vi "Write Image Header.vi"(8 "error in (no error)":errorcluster, 11 "Save Image in":refnum<class "Save Image.lvclass">) -> (0 "error out":errorcluster, 3 "Save Image out":refnum<class "Save Image.lvclass">)   [LabVIEW 2018, in "Save Image.lvclass"]
uses:
  Save Image.lvclass
  Save Image.lvclass/Save Image.ctl
  <userlib>/gfitsio/gfitsio-write-key-string.vi
  <userlib>/gfitsio/gfitsio.lvlib
  Simulated_Header/Simulated_Header.lvclass
panel:
  out "Header Contents":T1={"Header Content"={"FILENAME"={"Name"="FILENAME", "Value"="", "Comment"="File name at acquisition"}, "OBSERVER"={"Name"="OBSERVER", "Value"="", "Comment"="Name of the observer"}, "PROGRID"={"Name"="PROGRID", "Value"="", "Comment"="Program ID"}, "OBJECT"={"Name"="OBJECT", "Value"="", "Comment"="Object name"}, "NIGHTDIR"={"Name"="NIGHTDIR", "Value"="", "Comment"="Night directory name "}, "CHANNEL"={"Name"="CHANNEL", "Value"="", "Comment"="Instrument channel"}, "INSTRUME"={"Name"="INSTRUME", "Value"="", "Comment"="Instrument"}, "NEXPSEQ"={"Name"="NEXPSEQ", "Value"="", "Comment"="Total number of exposures in sequence"}, "SEQINDEX"={"Name"="SEQINDEX", "Value"="", "Comment"="Exposure index in the sequence"}, "OBSTYPE"={"Name"="OBSTYPE", "Value"="", "Comment"="Image type: OBJECT, BIAS, FLAT, ARC, DARK"}, "READMOD"={"Name"="READMOD", "Value"="", "Comment"="Read out mode: fast, normal, slow"}, "READMODE"={"Name"="READMODE", "Value"="", "Comment"="CCD read mode"}, "ACQMODE"={"Name"="ACQMODE", "Value"="", "Comment"="Acquisition Mode"}, "PREAMP"={"Name"="PREAMP", "Value"="", "Comment"="Pre-amplifier gain"}, "READOUT"={"Name"="READOUT", "Value"="", "Comment"="Readout Rate"}, "VSHIFT"={"Name"="VSHIFT", "Value"="", "Comment"="Vertical Shift Speed"}, "TRIGGER"={"Name"="TRIGGER", "Value"="", "Comment"="Trigger Mode"}, "EMMODE"={"Name"="EMMODE", "Value"="", "Comment"="Output amplifier mode"}, "EMGAIN"={"Name"="EMGAIN", "Value"="", "Comment"="EM Gain"}, "VBIN"={"Name"="VBIN", "Value"="", "Comment"="Vertical binning"}, "HBIN"={"Name"="HBIN", "Value"="", "Comment"="Horizontal binning"}, "INITLIN"={"Name"="INITLIN", "Value"="", "Comment"="Initial Line"}, "INITCOL"={"Name"="INITCOL", "Value"="", "Comment"="Initial Column"}, "FINALLIN"={"Name"="FINALLIN", "Value"="", "Comment"="Final Line"}, "FINALCOL"={"Name"="FINALCOL", "Value"="", "Comment"="Final Column"}, "KSERLEN"={"Name"="KSERLEN", "Value"="", "Comment"="Kinetic Series Length"}, "SHUTTER"={"Name"="SHUTTER", "Value"="", "Comment"="Shutter Mode (OPEN, CLOSED, or AUTO) "}, "OPENSHT"={"Name"="OPENSHT", "Value"="", "Comment"="Time to open the shutter (ms) "}, "CLOSESHT"={"Name"="CLOSESHT", "Value"="", "Comment"="Time to close the shutter (ms)"}, "DATE"={"Name"="DATE", "Value"="", "Comment"="Date of the acquired image (YY/MM/DD:HH:MM:SS.sss"}, "GAIN"={"Name"="GAIN", "Value"="", "Comment"="Gain (e-/ADU)"}, "GAINERR"={"Name"="GAINERR", "Value"="", "Comment"=" Gain error (e-/ADU)"}, "RDNOISE"={"Name"="RDNOISE", "Value"="", "Comment"="Read noise (e-)"}, "RNOISERR"={"Name"="RNOISERR", "Value"="", "Comment"="Read noise error (e-)"}, "SKYFIBER"={"Name"="SKYFIBER", "Value"="", "Comment"="Sky fiber: ON or OFF"}, "CALFIBER"={"Name"="CALFIBER", "Value"="", "Comment"="Calibration Fiber: ON or OFF"}, "UTDATE"={"Name"="UTDATE", "Value"="", "Comment"="UT date at start of exposure"}, "LOCTIME"={"Name"="LOCTIME", "Value"="", "Comment"="LT date at start of exposure"}, "MJD"={"Name"="MJD", "Value"="", "Comment"="Modified Julian Date at start of exposure"}, "OBSLON"={"Name"="OBSLON", "Value"="", "Comment"="Observatory East Longitude"}, "OBSLAT"={"Name"="OBSLAT", "Value"="", "Comment"="Observatory Latitude"}, "OBSALT"={"Name"="OBSALT", "Value"="", "Comment"="Observatory elevation above sea level (m)"}, "EXPTIME"={"Name"="EXPTIME", "Value"="", "Comment"="Exposure time (s)"}, "TELRA"={"Name"="TELRA", "Value"="", "Comment"="TCS right ascension: HH:MM:SS.SSS"}, "TELDEC"={"Name"="TELDEC", "Value"="", "Comment"="TCS declination: +-DD:MM:SS.SSS"}, "RA"={"Name"="RA", "Value"="", "Comment"="Requested right Ascension: HH:MM:SS.SSS"}, "DEC"={"Name"="DEC", "Value"="", "Comment"="Requested Declination: +- DD:MM:SS.SSS"}, "RA_DEG"={"Name"="RA_DEG", "Value"="", "Comment"="Requested Right Ascension (deg)"}, "DEC_DEG"={"Name"="DEC_DEG", "Value"="", "Comment"="Requested Declination (deg)"}, "EPOCH"={"Name"="EPOCH", "Value"="", "Comment"="Epoch for Target coordinates"}, "HA"={"Name"="HA", "Value"="", "Comment"="Hour Angle (Sexagesimal)"}, "HAD"={"Name"="HAD", "Value"="", "Comment"="Hour Angle (deg)"}, "AIRMASS"={"Name"="AIRMASS", "Value"="", "Comment"="Mean airmass for the observation"}, "AMSTART"={"Name"="AMSTART", "Value"="", "Comment"="Airmass at start of exposure"}, "AMEND"={"Name"="AMEND", "Value"="", "Comment"="Airmass at end of exposure"}, "XOFFSET"={"Name"="XOFFSET", "Value"="", "Comment"="Telescope RA offset in arcsec"}, "YOFFSET"={"Name"="YOFFSET", "Value"="", "Comment"="Telescope DEC offset in arcsec"}, "PA"={"Name"="PA", "Value"="", "Comment"="Current Rotator Position Angle (degree)"}, "CAMFOC"={"Name"="CAMFOC", "Value"="", "Comment"="Camera focus position (mm)"}, "TELFOC"={"Name"="TELFOC", "Value"="", "Comment"="Telescope focus position (mm)"}, "TCSUT"={"Name"="TCSUT", "Value"="", "Comment"="TCS Universal Time"}, "TCSST"={"Name"="TCSST", "Value"="", "Comment"="TCS Sideral Time"}, "MOONDIST"={"Name"="MOONDIST", "Value"="", "Comment"="Moon angular distance to object (deg)"}, "MOONALT"={"Name"="MOONALT", "Value"="", "Comment"="Moon elevation above horizon (deg)"}, "MOONPHAS"={"Name"="MOONPHAS", "Value"="", "Comment"="Moon elevation above horizon (deg)"}, "ADC"={"Name"="ADC", "Value"="", "Comment"="Atmospheric Dispersion Corrector: ON or OFF"}, "ADCSPEED"={"Name"="ADCSPEED", "Value"="", "Comment"="ADC motor speed (rpm)"}, "CALMIRR"={"Name"="CALMIRR", "Value"="", "Comment"="Calibration mirror position: IN or OUT"}, "GUIDING"={"Name"="GUIDING", "Value"="", "Comment"="Guider status: ON or OFF"}, "GUIDTEXP"={"Name"="GUIDTEXP", "Value"="", "Comment"="Guider exposure time (s)"}, "GUIDFREQ"={"Name"="GUIDFREQ", "Value"="", "Comment"="Guiding frequency (Hz)"}, "GUIDOBJX"={"Name"="GUIDOBJX", "Value"="", "Comment"="Guiding object x position (pixel)"}, "GUIDOBJY"={"Name"="GUIDOBJY", "Value"="", "Comment"="Guiding object y position (pixel)"}, "AVGYCORR"={"Name"="AVGYCORR", "Value"="", "Comment"="Average correction in RA (arcsec)"}, "AVGXCORR"={"Name"="AVGXCORR", "Value"="", "Comment"="Average correction in DEC (arcsec)"}, "GFOCUS"={"Name"="GFOCUS", "Value"="", "Comment"="Guider focus position (mm)"}, "THARLAMP"={"Name"="THARLAMP", "Value"="", "Comment"="Thorium-Argon lamp state: ON or OFF"}, "HALLAMP"={"Name"="HALLAMP", "Value"="", "Comment"="Halogen lamp state: ON or OFF"}, "AGITATOR"={"Name"="AGITATOR", "Value"="", "Comment"="Fiber agitator: ON or OFF"}, "THARMIRR"={"Name"="THARMIRR", "Value"="", "Comment"="Th-Ar mirror position: SPECTROGRAPH or TELESCOPE"}, "DSTATUS"={"Name"="DSTATUS", "Value"="", "Comment"="Dome Status: OPEN or CLOSED"}, "DPOS"={"Name"="DPOS", "Value"="", "Comment"="Dome position (deg)"}, "DTEMP"={"Name"="DTEMP", "Value"="", "Comment"="Dome temperature (deg C)"}, "DHUM"={"Name"="DHUM", "Value"="", "Comment"="Dome humidity (per cent)"}, "DLAMP"={"Name"="DLAMP", "Value"="", "Comment"="Dome lamp: ON or OFF"}, "DFLAT"={"Name"="DFLAT", "Value"="", "Comment"="Dome flat lamp: ON or OFF"}, "TEMPEXT"={"Name"="TEMPEXT", "Value"="", "Comment"="External temperature (deg C)"}, "PRESSURE"={"Name"="PRESSURE", "Value"="", "Comment"="Pressure (mbar)"}, "HUMIDITY"={"Name"="HUMIDITY", "Value"="", "Comment"="Humidity (per cent)"}, "WINDDIR"={"Name"="WINDDIR", "Value"="", "Comment"="Wind direction: North-eastward (deg)"}, "WINSPEED"={"Name"="WINSPEED", "Value"="", "Comment"="Wind Speed (km/h)"}, "SHTTTL"={"Name"="SHTTTL", "Value"="", "Comment"="Shutter TTL"}, "COOLER"={"Name"="COOLER", "Value"="", "Comment"="CCD cooler: ON or OFF"}, "TEMP"={"Name"="TEMP", "Value"="", "Comment"="CCD temperature"}, "TEMPST"={"Name"="TEMPST", "Value"="", "Comment"="Temperature status"}, "SERN"={"Name"="SERN", "Value"="", "Comment"="Serial Number"}, "OBS_TITLE"={"Name"="OBSTITLE", "Value"="", "Comment"="Observation Title"}, "COMMENT"={"Name"="COMMENT", "Value"="", "Comment"="Observation comment"}, "SIMPLE"={"Name"="SIMPLE", "Value"="file does conform to FITS standard\nFile does conform to FITS standard\nfile does conform to FITS standard", "Comment"=""}, "BITPIX"={"Name"="BITPIX\nBITPIX\nBITPIX", "Value"="16", "Comment"="Number of bits per data pixel"}, "NAXIS"={"Name"="BITPIX\nBITPIX\nNAXIS\nNAXIS", "Value"="3", "Comment"="Number of data axes"}, "EXTEND"={"Name"="BITPIX\nBITPIX\nNAXIS\nEXTEND\nEXTEND", "Value"="FITS dataset may contain extensions", "Comment"=""}}, "Image Delays"=[], "Headers to be written"=[]}
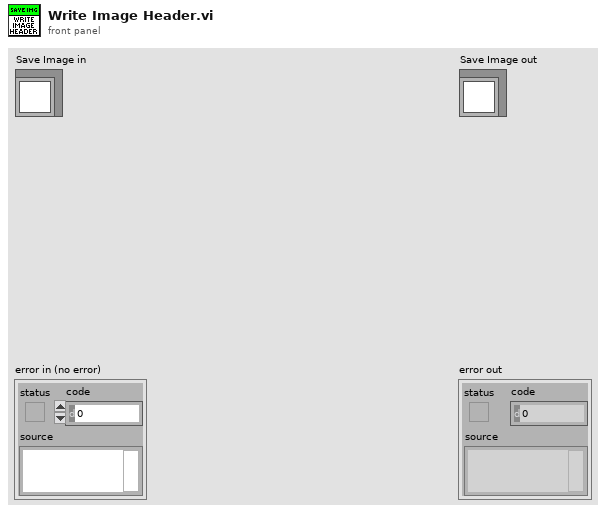
[diagram p1: front panel]
types:
  T1 = cluster{"Header Content":cluster{"FILENAME":cluster{"Name":string, "Value":string, "Comment":string}, "OBSERVER":cluster{"Name":string, "Value":string, "Comment":string}, "PROGRID":cluster{"Name":string, "Value":string, "Comment":string}, "OBJECT":cluster{"Name":string, "Value":string, "Comment":string}, "NIGHTDIR":cluster{"Name":string, "Value":string, "Comment":string}, "CHANNEL":cluster{"Name":string, "Value":string, "Comment":string}, "INSTRUME":cluster{"Name":string, "Value":string, "Comment":string}, "NEXPSEQ":cluster{"Name":string, "Value":string, "Comment":string}, "SEQINDEX":cluster{"Name":string, "Value":string, "Comment":string}, "OBSTYPE":cluster{"Name":string, "Value":string, "Comment":string}, "READMOD":cluster{"Name":string, "Value":string, "Comment":string}, "READMODE":cluster{"Name":string, "Value":string, "Comment":string}, "ACQMODE":cluster{"Name":string, "Value":string, "Comment":string}, "PREAMP":cluster{"Name":string, "Value":string, "Comment":string}, "READOUT":cluster{"Name":string, "Value":string, "Comment":string}, "VSHIFT":cluster{"Name":string, "Value":string, "Comment":string}, "TRIGGER":cluster{"Name":string, "Value":string, "Comment":string}, "EMMODE":cluster{"Name":string, "Value":string, "Comment":string}, "EMGAIN":cluster{"Name":string, "Value":string, "Comment":string}, "VBIN":cluster{"Name":string, "Value":string, "Comment":string}, "HBIN":cluster{"Name":string, "Value":string, "Comment":string}, "INITLIN":cluster{"Name":string, "Value":string, "Comment":string}, "INITCOL":cluster{"Name":string, "Value":string, "Comment":string}, "FINALLIN":cluster{"Name":string, "Value":string, "Comment":string}, "FINALCOL":cluster{"Name":string, "Value":string, "Comment":string}, "KSERLEN":cluster{"Name":string, "Value":string, "Comment":string}, "SHUTTER":cluster{"Name":string, "Value":string, "Comment":string}, "OPENSHT":cluster{"Name":string, "Value":string, "Comment":string}, "CLOSESHT":cluster{"Name":string, "Value":string, "Comment":string}, "DATE":cluster{"Name":string, "Value":string, "Comment":string}, "GAIN":cluster{"Name":string, "Value":string, "Comment":string}, "GAINERR":cluster{"Name":string, "Value":string, "Comment":string}, "RDNOISE":cluster{"Name":string, "Value":string, "Comment":string}, "RNOISERR":cluster{"Name":string, "Value":string, "Comment":string}, "SKYFIBER":cluster{"Name":string, "Value":string, "Comment":string}, "CALFIBER":cluster{"Name":string, "Value":string, "Comment":string}, "UTDATE":cluster{"Name":string, "Value":string, "Comment":string}, "LOCTIME":cluster{"Name":string, "Value":string, "Comment":string}, "MJD":cluster{"Name":string, "Value":string, "Comment":string}, "OBSLON":cluster{"Name":string, "Value":string, "Comment":string}, "OBSLAT":cluster{"Name":string, "Value":string, "Comment":string}, "OBSALT":cluster{"Name":string, "Value":string, "Comment":string}, "EXPTIME":cluster{"Name":string, "Value":string, "Comment":string}, "TELRA":cluster{"Name":string, "Value":string, "Comment":string}, "TELDEC":cluster{"Name":string, "Value":string, "Comment":string}, "RA":cluster{"Name":string, "Value":string, "Comment":string}, "DEC":cluster{"Name":string, "Value":string, "Comment":string}, "RA_DEG":cluster{"Name":string, "Value":string, "Comment":string}, "DEC_DEG":cluster{"Name":string, "Value":string, "Comment":string}, "EPOCH":cluster{"Name":string, "Value":string, "Comment":string}, "HA":cluster{"Name":string, "Value":string, "Comment":string}, "HAD":cluster{"Name":string, "Value":string, "Comment":string}, "AIRMASS":cluster{"Name":string, "Value":string, "Comment":string}, "AMSTART":cluster{"Name":string, "Value":string, "Comment":string}, "AMEND":cluster{"Name":string, "Value":string, "Comment":string}, "XOFFSET":cluster{"Name":string, "Value":string, "Comment":string}, "YOFFSET":cluster{"Name":string, "Value":string, "Comment":string}, "PA":cluster{"Name":string, "Value":string, "Comment":string}, "CAMFOC":cluster{"Name":string, "Value":string, "Comment":string}, "TELFOC":cluster{"Name":string, "Value":string, "Comment":string}, "TCSUT":cluster{"Name":string, "Value":string, "Comment":string}, "TCSST":cluster{"Name":string, "Value":string, "Comment":string}, "MOONDIST":cluster{"Name":string, "Value":string, "Comment":string}, "MOONALT":cluster{"Name":string, "Value":string, "Comment":string}, "MOONPHAS":cluster{"Name":string, "Value":string, "Comment":string}, "ADC":cluster{"Name":string, "Value":string, "Comment":string}, "ADCSPEED":cluster{"Name":string, "Value":string, "Comment":string}, "CALMIRR":cluster{"Name":string, "Value":string, "Comment":string}, "GUIDING":cluster{"Name":string, "Value":string, "Comment":string}, "GUIDTEXP":cluster{"Name":string, "Value":string, "Comment":string}, "GUIDFREQ":cluster{"Name":string, "Value":string, "Comment":string}, "GUIDOBJX":cluster{"Name":string, "Value":string, "Comment":string}, "GUIDOBJY":cluster{"Name":string, "Value":string, "Comment":string}, "AVGYCORR":cluster{"Name":string, "Value":string, "Comment":string}, "AVGXCORR":cluster{"Name":string, "Value":string, "Comment":string}, "GFOCUS":cluster{"Name":string, "Value":string, "Comment":string}, "THARLAMP":cluster{"Name":string, "Value":string, "Comment":string}, "HALLAMP":cluster{"Name":string, "Value":string, "Comment":string}, "AGITATOR":cluster{"Name":string, "Value":string, "Comment":string}, "THARMIRR":cluster{"Name":string, "Value":string, "Comment":string}, "DSTATUS":cluster{"Name":string, "Value":string, "Comment":string}, "DPOS":cluster{"Name":string, "Value":string, "Comment":string}, "DTEMP":cluster{"Name":string, "Value":string, "Comment":string}, "DHUM":cluster{"Name":string, "Value":string, "Comment":string}, "DLAMP":cluster{"Name":string, "Value":string, "Comment":string}, "DFLAT":cluster{"Name":string, "Value":string, "Comment":string}, "TEMPEXT":cluster{"Name":string, "Value":string, "Comment":string}, "PRESSURE":cluster{"Name":string, "Value":string, "Comment":string}, "HUMIDITY":cluster{"Name":string, "Value":string, "Comment":string}, "WINDDIR":cluster{"Name":string, "Value":string, "Comment":string}, "WINSPEED":cluster{"Name":string, "Value":string, "Comment":string}, "SHTTTL":cluster{"Name":string, "Value":string, "Comment":string}, "COOLER":cluster{"Name":string, "Value":string, "Comment":string}, "TEMP":cluster{"Name":string, "Value":string, "Comment":string}, "TEMPST":cluster{"Name":string, "Value":string, "Comment":string}, "SERN":cluster{"Name":string, "Value":string, "Comment":string}, "OBS_TITLE":cluster{"Name":string, "Value":string, "Comment":string}, "COMMENT":cluster{"Name":string, "Value":string, "Comment":string}, "SIMPLE":cluster{"Name":string, "Value":string, "Comment":string}, "BITPIX":cluster{"Name":string, "Value":string, "Comment":string}, "NAXIS":cluster{"Name":string, "Value":string, "Comment":string}, "EXTEND":cluster{"Name":string, "Value":string, "Comment":string}}, "Image Delays":string[], "Headers to be written":string[][]}
  T2 = enum16{"open", "open or create", "create or replace", "create", "open (read only)"}
  T3 = cluster{"Name":string, "Value":string, "Comment":string}
  T4 = typedef "gfitsio.lvlib/gfitsio-refnum.ctl" = refnum<k1>
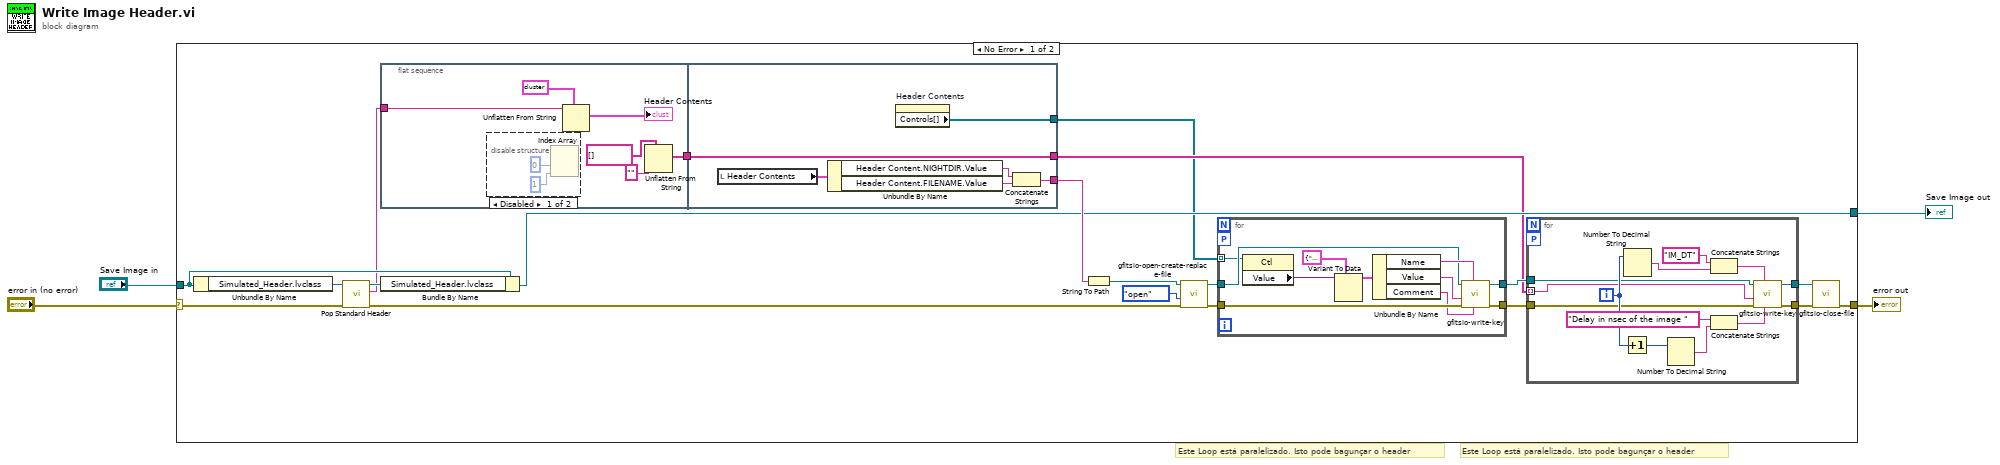
[diagram p0: block diagram]
diagram:
  # "Este Loop está paralelizado. Isto pode bagunçar o header"
  # "Este Loop está paralelizado. Isto pode bagunçar o header"
  n1 = case shown="No Error" "error in (no error)" {
    selector: "error in (no error)" -> [w10 w64]
    tunnel: [w24 w64] -> w3
    tunnel: [w13 w63] -> w1
    tunnel: "Save Image in" -> [w14 w63]
    frame No Error {
      n2 = Unbundle By Name(w14) -> ("Simulated_Header.lvclass"=w8:refnum<class "Simulated_Header.lvclass">)
      n3 = call "Pop Standard Header.vi"("error in (no error)"=w10, "Header in"=w8) -> ("error out"=w9:errorcluster, "Std Header"=w6:string, "Header out"=w7:refnum<class "Simulated_Header.lvclass">)  [unwired: 7 in]
      n4 = flat-sequence {
        tunnel: w6 -> [w26]
        tunnel: [w29] -> w11
        tunnel: [w38] -> w15
        tunnel: [w37] -> w12
        tunnel: w11 -> [w37]
        tunnel: [w33] -> w5
        frame #0 {
          n5 = disable-structure shown="Disabled" {
            frame Disabled {
              n6 = Index Array(index #1=0 ("disabled index (col)"), index #2=1 ("disabled index (col)")) -> ()  [unwired: 1 in, 2 out]
            }
            frame Enabled {
            }
          }
          n7 = Unflatten From String(type=T1 {"Header Content"={"FILENAME"={"Name"="FILENAME", "Value"="", "Comment"="File name at acquisition"}, "OBSERVER"={"Name"="OBSERVER", "Value"="", "Comment"="Name of the observer"}, "PROGRID"={"Name"="PROGRID", "Value"="", "Comment"="Program ID"}, "OBJECT"={"Name"="OBJECT", "Value"="", "Comment"="Object name"}, "NIGHTDIR"={"Name"="NIGHTDIR", "Value"="", "Comment"="Night directory name "}, "CHANNEL"={"Name"="CHANNEL", "Value"="", "Comment"="Instrument channel"}, "INSTRUME"={"Name"="INSTRUME", "Value"="", "Comment"="Instrument"}, "NEXPSEQ"={"Name"="NEXPSEQ", "Value"="", "Comment"="Total number of exposures in sequence"}, "SEQINDEX"={"Name"="SEQINDEX", "Value"="", "Comment"="Exposure index in the sequence"}, "OBSTYPE"={"Name"="OBSTYPE", "Value"="", "Comment"="Image type: OBJECT, BIAS, FLAT, ARC, DARK"}, "READMOD"={"Name"="READMOD", "Value"="", "Comment"="Read out mode: fast, normal, slow"}, "READMODE"={"Name"="READMODE", "Value"="", "Comment"="CCD read mode"}, "ACQMODE"={"Name"="ACQMODE", "Value"="", "Comment"="Acquisition Mode"}, "PREAMP"={"Name"="PREAMP", "Value"="", "Comment"="Pre-amplifier gain"}, "READOUT"={"Name"="READOUT", "Value"="", "Comment"="Readout Rate"}, "VSHIFT"={"Name"="VSHIFT", "Value"="", "Comment"="Vertical Shift Speed"}, "TRIGGER"={"Name"="TRIGGER", "Value"="", "Comment"="Trigger Mode"}, "EMMODE"={"Name"="EMMODE", "Value"="", "Comment"="Output amplifier mode"}, "EMGAIN"={"Name"="EMGAIN", "Value"="", "Comment"="EM Gain"}, "VBIN"={"Name"="VBIN", "Value"="", "Comment"="Vertical binning"}, "HBIN"={"Name"="HBIN", "Value"="", "Comment"="Horizontal binning"}, "INITLIN"={"Name"="INITLIN", "Value"="", "Comment"="Initial Line"}, "INITCOL"={"Name"="INITCOL", "Value"="", "Comment"="Initial Column"}, "FINALLIN"={"Name"="FINALLIN", "Value"="", "Comment"="Final Line"}, "FINALCOL"={"Name"="FINALCOL", "Value"="", "Comment"="Final Column"}, "KSERLEN"={"Name"="KSERLEN", "Value"="", "Comment"="Kinetic Series Length"}, "SHUTTER"={"Name"="SHUTTER", "Value"="", "Comment"="Shutter Mode (OPEN, CLOSED, or AUTO) "}, "OPENSHT"={"Name"="OPENSHT", "Value"="", "Comment"="Time to open the shutter (ms) "}, "CLOSESHT"={"Name"="CLOSESHT", "Value"="", "Comment"="Time to close the shutter (ms)"}, "DATE"={"Name"="DATE", "Value"="", "Comment"="Date of the acquired image (YY/MM/DD:HH:MM:SS.sss"}, "GAIN"={"Name"="GAIN", "Value"="", "Comment"="Gain (e-/ADU)"}, "GAINERR"={"Name"="GAINERR", "Value"="", "Comment"=" Gain error (e-/ADU)"}, "RDNOISE"={"Name"="RDNOISE", "Value"="", "Comment"="Read noise (e-)"}, "RNOISERR"={"Name"="RNOISERR", "Value"="", "Comment"="Read noise error (e-)"}, "SKYFIBER"={"Name"="SKYFIBER", "Value"="", "Comment"="Sky fiber: ON or OFF"}, "CALFIBER"={"Name"="CALFIBER", "Value"="", "Comment"="Calibration Fiber: ON or OFF"}, "UTDATE"={"Name"="UTDATE", "Value"="", "Comment"="UT date at start of exposure"}, "LOCTIME"={"Name"="LOCTIME", "Value"="", "Comment"="LT date at start of exposure"}, "MJD"={"Name"="MJD", "Value"="", "Comment"="Modified Julian Date at start of exposure"}, "OBSLON"={"Name"="OBSLON", "Value"="", "Comment"="Observatory East Longitude"}, "OBSLAT"={"Name"="OBSLAT", "Value"="", "Comment"="Observatory Latitude"}, "OBSALT"={"Name"="OBSALT", "Value"="", "Comment"="Observatory elevation above sea level (m)"}, "EXPTIME"={"Name"="EXPTIME", "Value"="", "Comment"="Exposure time (s)"}, "TELRA"={"Name"="TELRA", "Value"="", "Comment"="TCS right ascension: HH:MM:SS.SSS"}, "TELDEC"={"Name"="TELDEC", "Value"="", "Comment"="TCS declination: +-DD:MM:SS.SSS"}, "RA"={"Name"="RA", "Value"="", "Comment"="Requested right Ascension: HH:MM:SS.SSS"}, "DEC"={"Name"="DEC", "Value"="", "Comment"="Requested Declination: +- DD:MM:SS.SSS"}, "RA_DEG"={"Name"="RA_DEG", "Value"="", "Comment"="Requested Right Ascension (deg)"}, "DEC_DEG"={"Name"="DEC_DEG", "Value"="", "Comment"="Requested Declination (deg)"}, "EPOCH"={"Name"="EPOCH", "Value"="", "Comment"="Epoch for Target coordinates"}, "HA"={"Name"="HA", "Value"="", "Comment"="Hour Angle (Sexagesimal)"}, "HAD"={"Name"="HAD", "Value"="", "Comment"="Hour Angle (deg)"}, "AIRMASS"={"Name"="AIRMASS", "Value"="", "Comment"="Mean airmass for the observation"}, "AMSTART"={"Name"="AMSTART", "Value"="", "Comment"="Airmass at start of exposure"}, "AMEND"={"Name"="AMEND", "Value"="", "Comment"="Airmass at end of exposure"}, "XOFFSET"={"Name"="XOFFSET", "Value"="", "Comment"="Telescope RA offset in arcsec"}, "YOFFSET"={"Name"="YOFFSET", "Value"="", "Comment"="Telescope DEC offset in arcsec"}, "PA"={"Name"="PA", "Value"="", "Comment"="Current Rotator Position Angle (degree)"}, "CAMFOC"={"Name"="CAMFOC", "Value"="", "Comment"="Camera focus position (mm)"}, "TELFOC"={"Name"="TELFOC", "Value"="", "Comment"="Telescope focus position (mm)"}, "TCSUT"={"Name"="TCSUT", "Value"="", "Comment"="TCS Universal Time"}, "TCSST"={"Name"="TCSST", "Value"="", "Comment"="TCS Sideral Time"}, "MOONDIST"={"Name"="MOONDIST", "Value"="", "Comment"="Moon angular distance to object (deg)"}, "MOONALT"={"Name"="MOONALT", "Value"="", "Comment"="Moon elevation above horizon (deg)"}, "MOONPHAS"={"Name"="MOONPHAS", "Value"="", "Comment"="Moon elevation above horizon (deg)"}, "ADC"={"Name"="ADC", "Value"="", "Comment"="Atmospheric Dispersion Corrector: ON or OFF"}, "ADCSPEED"={"Name"="ADCSPEED", "Value"="", "Comment"="ADC motor speed (rpm)"}, "CALMIRR"={"Name"="CALMIRR", "Value"="", "Comment"="Calibration mirror position: IN or OUT"}, "GUIDING"={"Name"="GUIDING", "Value"="", "Comment"="Guider status: ON or OFF"}, "GUIDTEXP"={"Name"="GUIDTEXP", "Value"="", "Comment"="Guider exposure time (s)"}, "GUIDFREQ"={"Name"="GUIDFREQ", "Value"="", "Comment"="Guiding frequency (Hz)"}, "GUIDOBJX"={"Name"="GUIDOBJX", "Value"="", "Comment"="Guiding object x position (pixel)"}, "GUIDOBJY"={"Name"="GUIDOBJY", "Value"="", "Comment"="Guiding object y position (pixel)"}, "AVGYCORR"={"Name"="AVGYCORR", "Value"="", "Comment"="Average correction in RA (arcsec)"}, "AVGXCORR"={"Name"="AVGXCORR", "Value"="", "Comment"="Average correction in DEC (arcsec)"}, "GFOCUS"={"Name"="GFOCUS", "Value"="", "Comment"="Guider focus position (mm)"}, "THARLAMP"={"Name"="THARLAMP", "Value"="", "Comment"="Thorium-Argon lamp state: ON or OFF"}, "HALLAMP"={"Name"="HALLAMP", "Value"="", "Comment"="Halogen lamp state: ON or OFF"}, "AGITATOR"={"Name"="AGITATOR", "Value"="", "Comment"="Fiber agitator: ON or OFF"}, "THARMIRR"={"Name"="THARMIRR", "Value"="", "Comment"="Th-Ar mirror position: SPECTROGRAPH or TELESCOPE"}, "DSTATUS"={"Name"="DSTATUS", "Value"="", "Comment"="Dome Status: OPEN or CLOSED"}, "DPOS"={"Name"="DPOS", "Value"="", "Comment"="Dome position (deg)"}, "DTEMP"={"Name"="DTEMP", "Value"="", "Comment"="Dome temperature (deg C)"}, "DHUM"={"Name"="DHUM", "Value"="", "Comment"="Dome humidity (per cent)"}, "DLAMP"={"Name"="DLAMP", "Value"="", "Comment"="Dome lamp: ON or OFF"}, "DFLAT"={"Name"="DFLAT", "Value"="", "Comment"="Dome flat lamp: ON or OFF"}, "TEMPEXT"={"Name"="TEMPEXT", "Value"="", "Comment"="External temperature (deg C)"}, "PRESSURE"={"Name"="PRESSURE", "Value"="", "Comment"="Pressure (mbar)"}, "HUMIDITY"={"Name"="HUMIDITY", "Value"="", "Comment"="Humidity (per cent)"}, "WINDDIR"={"Name"="WINDDIR", "Value"="", "Comment"="Wind direction: North-eastward (deg)"}, "WINSPEED"={"Name"="WINSPEED", "Value"="", "Comment"="Wind Speed (km/h)"}, "SHTTTL"={"Name"="SHTTTL", "Value"="", "Comment"="Shutter TTL"}, "COOLER"={"Name"="COOLER", "Value"="", "Comment"="CCD cooler: ON or OFF"}, "TEMP"={"Name"="TEMP", "Value"="", "Comment"="CCD temperature"}, "TEMPST"={"Name"="TEMPST", "Value"="", "Comment"="Temperature status"}, "SERN"={"Name"="SERN", "Value"="", "Comment"="Serial Number"}, "OBS_TITLE"={"Name"="OBSTITLE", "Value"="", "Comment"="Observation Title"}, "COMMENT"={"Name"="COMMENT", "Value"="", "Comment"="Observation comment"}, "SIMPLE"={"Name"="SIMPLE", "Value"="file does conform to FITS standard\nFile does conform to FITS standard\nfile does conform to FITS standard", "Comment"=""}, "BITPIX"={"Name"="BITPIX\nBITPIX\nBITPIX", "Value"="16", "Comment"="Number of bits per data pixel"}, "NAXIS"={"Name"="BITPIX\nBITPIX\nNAXIS\nNAXIS", "Value"="3", "Comment"="Number of data axes"}, "EXTEND"={"Name"="BITPIX\nBITPIX\nNAXIS\nEXTEND\nEXTEND", "Value"="FITS dataset may contain extensions", "Comment"=""}}, "Image Delays"=[], "Headers to be written"=[]} ("Cluster of class private data 2"), binary string=w26) -> (value=→"Header Contents":T1)  [unwired: 3 in, 2 out]
          n8 = Unflatten From String(type=string[] [] ("Image Delays"), binary string="") -> (value=w29:string[])  [unwired: 3 in, 2 out]
        }
        frame #1 {
          n9 = local read "Header Contents"() -> (w34:T1)
          n10 = Unbundle By Name(w34) -> ("Header Content.NIGHTDIR.Value"=w36:string, "Header Content.FILENAME.Value"=w35:string)
          n11 = property on="Header Contents" class="Clust (strict)"() -> ("Controls[]"=w33:refnum<vi>[])  [unwired: 2 in, 2 out]
          n12 = Concatenate Strings(w36, w35) -> (w38:string)
        }
      }
      n13 = Bundle By Name(cluster=w14, "Simulated_Header.lvclass"=w7) -> (w13:refnum<class "Save Image.lvclass">)
      n14 = String To Path(string=w15) -> (path=w17:path)
      n15 = call <userlib>:"gfitsio-open-create-replace-file.vi"("error in (no error)"=w9, "function (open)"=T2."open", "file path (dialog if empty)"=w17) -> ("error out"=w19:errorcluster, "gfits refnum"=w16:T4)  [unwired: 6 in, 1 out]
      n16 = for {
        tunnel: [w54] -> w22
        tunnel: w19 -> [w61]
        tunnel: [w62] -> w20
        workers-P: _ -> [_]
        tunnel: w16 -> [w53]
        tunnel: w5 -> [w52] mode=indexing
        n17 = property class="Ctl"(reference=w52) -> ("Value"=w60:variant)  [unwired: 1 in, 2 out]
        n18 = Variant To Data(type=T3 {"Name"="", "Value"="", "Comment"=""} ("SERN"), Variant=w60) -> (data=w58:T3)  [unwired: 1 in, 1 out]
        n19 = Unbundle By Name(w58) -> ("Name"=w57:string, "Value"=w56:string, "Comment"=w55:string)
        n20 = call-poly <userlib>:"gfitsio-write-key.vi"("comment"=w55, "keyname"=w57, "error in (no error)"=w61, "value"=w56, "gfits refnum"=w53) -> ("error out"=w62:errorcluster, "dup gfits refnum"=w54:T4)  [unwired: 5 in]
      }
      n21 = for {
        tunnel: w22 -> [w41]
        tunnel: [w40] -> w21
        tunnel: w20 -> [w45]
        tunnel: [w44] -> w23
        workers-P: _ -> [_]
        tunnel: w12 -> [w39] mode=indexing
        i -> [w47]
        n22 = Increment(x=w47) -> (x+1=w48:i32)
        n23 = Number To Decimal String(number=w47) -> (decimal integer string=w50:string)  [unwired: 1 in]
        n24 = Number To Decimal String(number=w48) -> (decimal integer string=w42:string)  [unwired: 1 in]
        n25 = Concatenate Strings("IM_DT", w50) -> (w49:string)
        n26 = Concatenate Strings("Delay in nsec of the image " ("comment"), w42) -> (w46:string)
        n27 = call-poly <userlib>:"gfitsio-write-key.vi"("comment"=w46, "keyname"=w49, "error in (no error)"=w45, "value"=w39, "gfits refnum"=w41) -> ("error out"=w44:errorcluster, "dup gfits refnum"=w40:T4)  [unwired: 5 in]
      }
      n28 = call <userlib>:"gfitsio-close-file.vi"("error in (no error)"=w23, "gfits refnum"=w21) -> ("error out"=w24:errorcluster)  [unwired: 8 in, 1 out]
    }
    frame Error {
    }
  }
  "error out" <- w3
  "Save Image out" <- w1
